vi "Enable Disable Routing Channel RTM.vi"(8 "error in (no error)":errorcluster, 11 "Node Ptr":u64 format="%.0x") -> (0 "error out":errorcluster)   [LabVIEW 2020, in "Routing and Faulting System Explorer.lvlib"]
uses:
  Routing and Faulting System Explorer.lvlib
  <vilib>/NI VeriStand/Custom Device API/Custom Device API.lvlib
  <vilib>/NI VeriStand/Custom Device Tools/Custom Device Utility Library/Custom Device Utility Library.lvlib
panel:
  in  "Tag":string
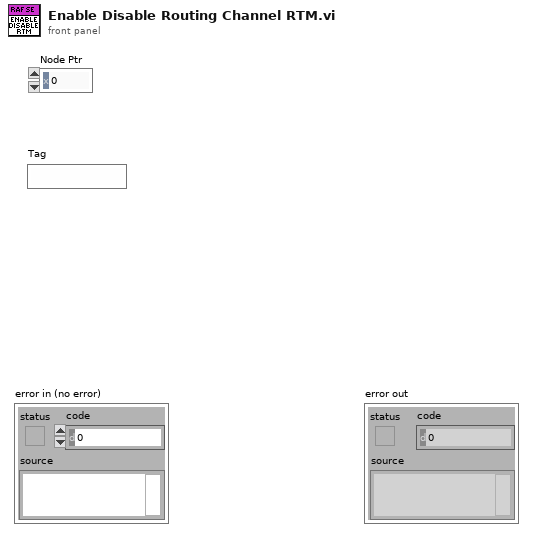
[diagram p1: front panel]
types:
  T1 = typedef "Custom Device API.lvlib/Custom Device Item Ref.ctl" = u64
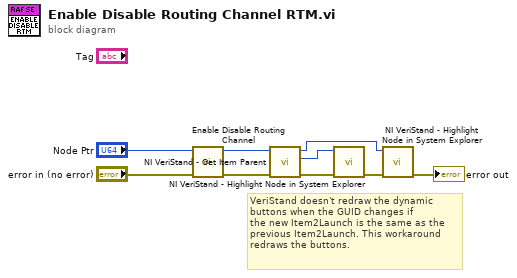
[diagram p0: block diagram]
diagram:
  # "VeriStand doesn't redraw the dynamic\nbuttons when the GUID changes if\nthe new Item2Launch is the same as the\nprevious Item2Launch. This workaround\nredraws the buttons."
  n1 = call "Enable Disable Routing Channel.vi"("error in (no error)"="error in (no error)", "Node Ptr"="Node Ptr") -> ("error out"=w2:errorcluster, "Node Ptr out"=w1:T1)  [unwired: 8 in]
  n2 = call <vilib>:"NI VeriStand - Get Item Parent.vi"("error in (no error)"=w2, "Item Ref in"=w1) -> ("error out"=w9:errorcluster, "Parent Ref"=w8:T1, "Item Ref out"=w6:T1)  [unwired: 6 in, 1 out]
  n3 = call <vilib>:"NI VeriStand - Highlight Node in System Explorer.vi"("error in (no error)"=w9, "Item Ref in"=w8) -> ("error out"=w7:errorcluster)  [unwired: 8 in, 1 out]
  n4 = call <vilib>:"NI VeriStand - Highlight Node in System Explorer.vi"("error in (no error)"=w7, "Item Ref in"=w6) -> ("error out"=→"error out":errorcluster)  [unwired: 8 in, 1 out]
